vi "Diamond Target Analysis.vi"(11 "Diamond Targets":T3[](array[typedef])) -> (3 "Targetting Output":T2)   [LabVIEW 2011]
uses:
  Diamond Target Output.ctl
  Rectangle Position.ctl
  Target Confidence.ctl
  Camera State.ctl
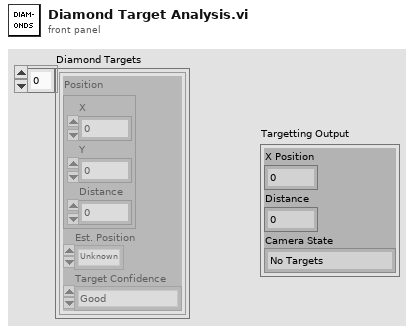
[diagram p1: front panel]
types:
  T1 = typedef "Camera State.ctl" = enum16{"No Targets", "Low Confidence", "Medium Confidence", "High Confidence", "Camera Error"}
  T2 = cluster{"X Position":dbl, "Distance":dbl, "Camera State":T1}
  T3 = typedef "Diamond Target Output.ctl" = cluster{"Position":cluster{"X":dbl, "Y":dbl, "Distance":dbl}, "Est. Position":T4, "Target Confidence":T5}
  T4 = typedef "Rectangle Position.ctl" = enum16{"Unknown", "Top", "Right", "Left", "Bottom"}
  T5 = typedef "Target Confidence.ctl" = enum16{"Good", "Good-Clipped Y", "Marginal-Clipped X"}
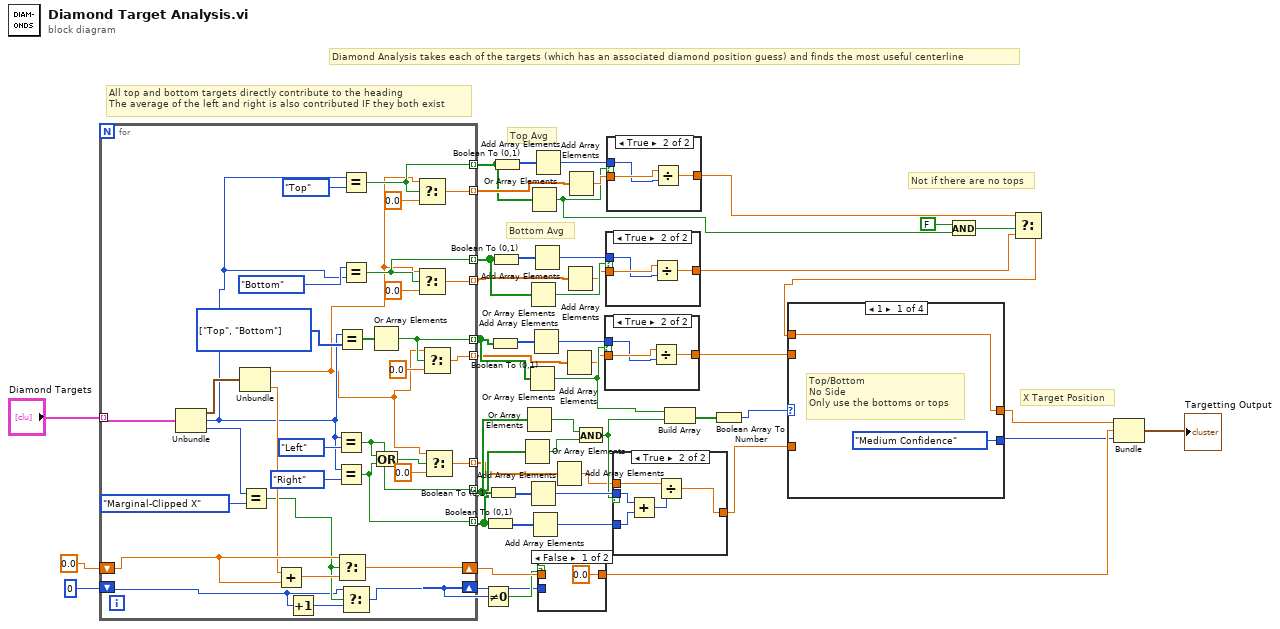
[diagram p0: block diagram]
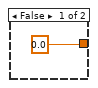
[diagram p2: hidden frame]
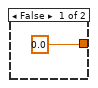
[diagram p3: hidden frame]
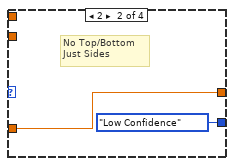
[diagram p4: hidden frame]
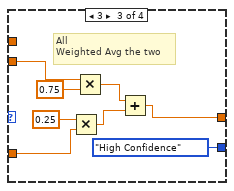
[diagram p5: hidden frame]
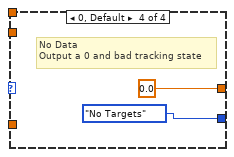
[diagram p6: hidden frame]
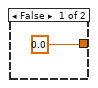
[diagram p7: hidden frame]
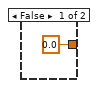
[diagram p8: hidden frame]
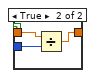
[diagram p9: hidden frame]
diagram:
  # "Diamond Analysis takes each of the targets (which has an associated diamond position guess) and finds the most useful centerline"
  # "Not if there are no tops"
  # "Top Avg"
  # "Bottom Avg"
  # "X Target Position"
  # "All top and bottom targets directly contribute to the heading\nThe average of the left and right is also contributed IF they both exist"
  n1 = for {
    tunnel: "Diamond Targets" -> [w82] mode=indexing
    tunnel: [w65] -> w34 mode=indexing
    tunnel: [w63] -> w36 mode=indexing
    shift-right: [w74] -> w45
    shift-left: 0.0 -> [w72]
    shift-right: [w70] -> w43
    shift-left: 0 -> [w67]
    tunnel: [w66] -> w35 mode=indexing
    tunnel: [w62] -> w22 mode=indexing
    tunnel: [w60] -> w20 mode=indexing
    tunnel: [w56] -> w12 mode=indexing
    tunnel: [w55] -> w13 mode=indexing
    tunnel: [w51] -> w8 mode=indexing
    tunnel: [w50] -> w7 mode=indexing
    w76 = T4[] [enum."Top", enum."Bottom"] items=["Unknown", "Top", "Right", "Left", "Bottom"]
    n2 = Unbundle(w82) -> ("Position"=w81:cluster{"X":dbl, "Y":dbl, "Distance":dbl}, "Est. Position"=w53:T4, "Target Confidence"=w80:T5)
    n3 = Unbundle(w81) -> ("X"=w49:dbl, "Distance"=w71:dbl)  [unwired: 1 out]
    n4 = Equal?(x=w80, y=Target_Confidence."Marginal-Clipped X") -> (x = y?=w69:bool)
    n5 = Add(x=w71, y=w72) -> (x+y=w73:dbl)
    n6 = Increment(x=w67) -> (x+1=w68:i32)
    n7 = Equal?(x=w53, y=Rectangle_Position."Left") -> (x = y?=w66:bool)
    n8 = Equal?(x=w53, y=Rectangle_Position."Right") -> (x = y?=w65:bool)
    n9 = Equal?(x=w53, y=w76) -> (x = y?=w75:bool[])
    n10 = Select(t=w72, s=w69, f=w73) -> (s? t:f=w74:dbl)
    n11 = Equal?(x=w53, y=Rectangle_Position."Top") -> (x = y?=w50:bool)
    n12 = Equal?(x=Rectangle_Position."Bottom" ("y"), y=w53) -> (x = y?=w55:bool)
    n13 = Select(t=w67, s=w69, f=w68) -> (s? t:f=w70:i32)
    n14 = Or Array Elements(Boolean array=w75) -> (logical OR=w63:bool)
    n15 = Or(x=w66, y=w65) -> (x .or. y?=w64:bool)
    n16 = Select(t=w49, s=w50, f=0.0) -> (s? t:f=w51:dbl)
    n17 = Select(t=w49, s=w55, f=0.0) -> (s? t:f=w56:dbl)
    n18 = Select(t=w49, s=w63, f=0.0) -> (s? t:f=w60:dbl)
    n19 = Select(t=w49, s=w64, f=0.0) -> (s? t:f=w62:dbl)
  }
  n20 = Not Equal To 0?(x=w43) -> (x != 0?=w44:bool)
  n21 = Boolean To (0,1)(Boolean=w34) -> (0, 1=w40:i16[])
  n22 = Boolean To (0,1)(Boolean=w35) -> (0, 1=w41:i16[])
  n23 = Boolean To (0,1)(Boolean=w36) -> (0, 1=w42:i16[])
  n24 = Boolean To (0,1)(Boolean=w13) -> (0, 1=w17:i16[])
  n25 = Boolean To (0,1)(Boolean=w7) -> (0, 1=w11:i16[])
  n26 = Or Array Elements(Boolean array=w34) -> (logical OR=w32:bool)
  n27 = Or Array Elements(Boolean array=w35) -> (logical OR=w33:bool)
  n28 = Or Array Elements(Boolean array=w36) -> (logical OR=w31:bool)
  n29 = Or Array Elements(Boolean array=w13) -> (logical OR=w15:bool)
  n30 = Add Array Elements(numeric array=w41) -> (sum=w38:i16)
  n31 = Or Array Elements(Boolean array=w7) -> (logical OR=w2:bool)
  n32 = Add Array Elements(numeric array=w40) -> (sum=w37:i16)
  n33 = Add Array Elements(numeric array=w42) -> (sum=w39:i16)
  n34 = Add Array Elements(numeric array=w17) -> (sum=w16:i16)
  n35 = Add Array Elements(numeric array=w11) -> (sum=w10:i16)
  n36 = case shown="False" w44 {
    tunnel: w45 -> [_ w86]
    tunnel: w43 -> [_ w85]
    tunnel: [0.0 w84] -> w24
    frame False {
    }
    frame True {
      n37 = Divide(x=w86, y=w85) -> (x/y=w84:dbl)
    }
  }
  n38 = Add Array Elements(numeric array=w22) -> (sum=w21:dbl)
  n39 = Add Array Elements(numeric array=w20) -> (sum=w19:dbl)
  n40 = Add Array Elements(numeric array=w12) -> (sum=w14:dbl)
  n41 = Add Array Elements(numeric array=w8) -> (sum=w9:dbl)
  n42 = And(x=w33, y=w32) -> (x .and. y?=w30:bool)
  n43 = case shown="True" w31 {
    tunnel: w19 -> [_ w90]
    tunnel: w39 -> [_ w89]
    tunnel: [0.0 w88] -> w27
    frame False {
    }
    frame True {
      n44 = Divide(x=w90, y=w89) -> (x/y=w88:dbl)
    }
  }
  n45 = case shown="True" w15 {
    tunnel: w14 -> [_ w94]
    tunnel: w16 -> [_ w93]
    tunnel: [0.0 w92] -> w5
    frame False {
    }
    frame True {
      n46 = Divide(x=w94, y=w93) -> (x/y=w92:dbl)
    }
  }
  n47 = case shown="True" w2 {
    tunnel: w9 -> [_ w98]
    tunnel: w10 -> [_ w97]
    tunnel: [0.0 w96] -> w6
    frame False {
    }
    frame True {
      n48 = Divide(x=w98, y=w97) -> (x/y=w96:dbl)
    }
  }
  n49 = case shown="True" w30 {
    tunnel: w38 -> [_ w104]
    tunnel: w37 -> [_ w103]
    tunnel: [0.0 w100] -> w26
    tunnel: w21 -> [_ w101]
    frame False {
    }
    frame True {
      n50 = Add(x=w104, y=w103) -> (x+y=w102:i16)
      n51 = Divide(x=w101, y=w102) -> (x/y=w100:dbl)
    }
  }
  n52 = Build Array(w31, w30) -> (w29:bool[])
  n53 = Boolean Array To Number(Boolean array=w29) -> (number=w28:u32)
  n54 = And(x=FALSE, y=w2) -> (x .and. y?=w3:bool)
  n55 = Select(t=w6, s=w3, f=w5) -> (s? t:f=w4:dbl)
  n56 = case shown="1" w28 {
    tunnel: [Camera_State."Medium Confidence" ("Camera State") Camera_State."Low Confidence" ("Camera State") Camera_State."High Confidence" ("Camera State") Camera_State."No Targets" ("Camera State")] -> w23
    tunnel: [w105 w107 w109 0.0] -> w25
    tunnel: w27 -> [_ _ w115 _]
    tunnel: w26 -> [_ w107 w112 _]
    tunnel: w4 -> [w105 _ _ _]
    frame 1 {
      # "Top/Bottom\nNo Side\nOnly use the bottoms or tops"
    }
    frame 2 {
      # "No Top/Bottom\nJust Sides"
    }
    frame 3 {
      # "All\nWeighted Avg the two"
      n57 = Multiply(x=0.25, y=w112) -> (x*y=w110:dbl)
      n58 = Multiply(x=w115, y=0.75) -> (x*y=w111:dbl)
      n59 = Add(x=w111, y=w110) -> (x+y=w109:dbl)
    }
    frame 0, Default {
      # "No Data\nOutput a 0 and bad tracking state"
    }
  }
  n60 = Bundle(w25, w24, "Camera State"=w23) -> (→"Targetting Output":cluster{dbl, dbl, "Camera State":T1})  [unwired: 1 in]
